vi "Redraw Window.vi"(8 "error in (no error)":errorcluster, 11 "Hwnd":u32) -> (0 "error out":errorcluster)   [LabVIEW 2011]
doc: "This VI will redraw the window provided by <b>Hwnd</b>."
uses:
  user32.dll
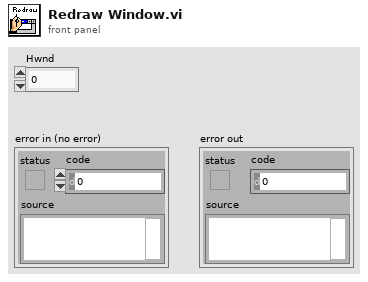
[diagram p1: front panel]
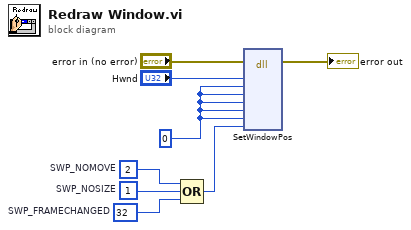
[diagram p0: block diagram]
diagram:
  w5 = u32 32  # SWP_FRAMECHANGED
  w4 = u32 1  # SWP_NOSIZE
  w3 = u32 2  # SWP_NOMOVE
  w2 = u32 0 ("arg2")
  n1 = Compound Arithmetic op=OR(w3, w4, w5) -> (w6:u32)
  n2 = dll-call lib="USER32.DLL" fn="SetWindowPos"(error in="error in (no error)", "hWnd"="Hwnd", "arg2"=w2, "left"=w2, "top"=w2, "right"=w2, "bottom"=w2, "Flags"=w6) -> (error out=→"error out":errorcluster)  [unwired: 4 in, 7 out]
